vi "SetExportType.vi"(8 "error in (no error)":errorcluster, 9 "Export type":T1, 11 "IExporter in":refnum<class "IExporter.lvclass">) -> (0 "error out":errorcluster, 3 "IExporter out":refnum<class "IExporter.lvclass">)   [LabVIEW 2020, in "ExtensionInterfaces.lvlib" / "IExporter.lvclass"]
uses:
  IExporter.lvclass
  ExportType.ctl
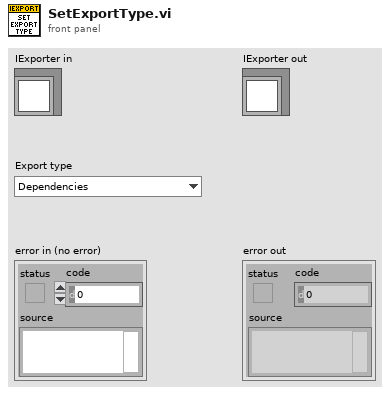
[diagram p1: front panel]
types:
  T1 = typedef "ExtensionInterfaces.lvlib/IExporter.lvclass/ExportType.ctl" = enum16{"Dependencies", "Rules", "Invalid dependencies", "Concessions", "Undeclared"}
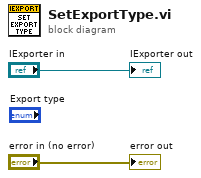
[diagram p0: block diagram]
diagram:
  "error out" <- "error in (no error)"
  "IExporter out" <- "IExporter in"
